vi "Avantes - AVS Init.vi"(8 "error in (no error)":errorcluster, 10 "a_Port":i32, 11 "Cluster in":T1) -> (0 "error out":errorcluster, 3 "Cluster out":T1)   [LabVIEW 2013, in "Avantes Spectrometer Functions.lvlib"]
uses:
  Avantes Spectrometer Functions.lvlib
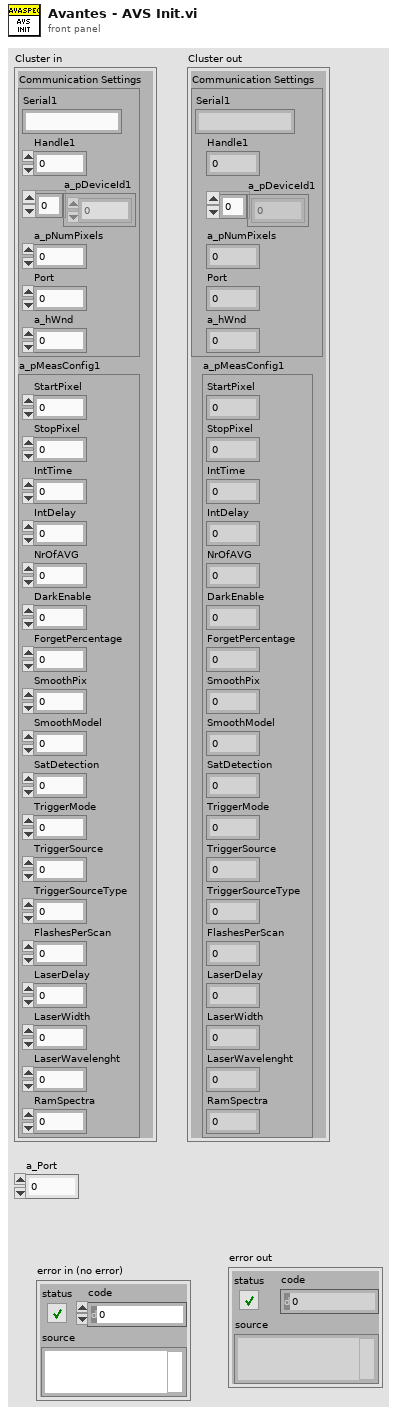
[diagram p1: front panel]
types:
  T1 = cluster{"Communication Settings":cluster{"Serial1":string, "Handle1":i32, "a_pDeviceId1":u8[], "a_pNumPixels":u16, "Port":i32, "a_hWnd":i32}, "a_pMeasConfig1":cluster{"StartPixel":u16, "StopPixel":u16, "IntTime":sgl, "IntDelay":u32, "NrOfAVG":u32, "DarkEnable":u8, "ForgetPercentage":u8, "SmoothPix":u16, "SmoothModel":u8, "SatDetection":u8, "TriggerMode":u8, "TriggerSource":u8, "TriggerSourceType":u8, "FlashesPerScan":u16, "LaserDelay":u32, "LaserWidth":u32, "LaserWavelenght":sgl, "RamSpectra":u16}}
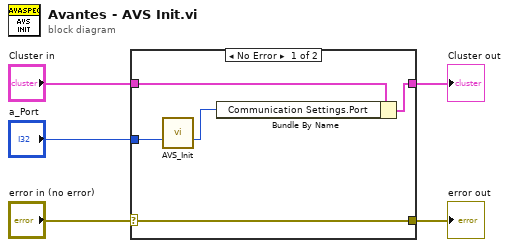
[diagram p0: block diagram]
diagram:
  n1 = case shown="No Error" "error in (no error)" {
    selector: "error in (no error)" -> [w6 w12]
    tunnel: [w10 w11] -> w5
    tunnel: "Cluster in" -> [w8 w11]
    tunnel: "a_Port" -> [w7 _]
    tunnel: [w6 w12] -> w1
    frame No Error {
      n2 = call "AVS_Init.vi"("a_Port"=w7) -> ("Output Value"=w9:i32)  [unwired: 14 in]
      n3 = Bundle By Name(cluster=w8, "Communication Settings.Port"=w9) -> (w10:T1)
    }
    frame Error {
    }
  }
  "Cluster out" <- w5
  "error out" <- w1
